vi "Main.Initialize DTC FIFOs.vi"(8 "error in":errorcluster, 11 "Sim DTCs":T2 {"DM1 Ref"."Data Reference" format="%.0x"; "DM1 Enable Ref"."Data Reference" format="%.0x"; "DM2 Ref"."Data Reference" format="%.0x"; "DM2 Enable Ref"."Data Reference" format="%.0x"}) -> (0 "error out":errorcluster, 3 "Sim DTC Refs":T1 {"Data"."DM1 Ref"."Data Reference" format="%.0x"; "Data"."DM1 Enable Ref"."Data Reference" format="%.0x"; "Data"."DM2 Ref"."Data Reference" format="%.0x"; "Data"."DM2 Enable Ref"."Data Reference" format="%.0x"})   [LabVIEW 2015, in "J1939 Addon Engine.lvlib"]
uses:
  J1939 Addon Engine.lvlib
  Shared/Types/Compiled Simulated Settings.ctl
  <vilib>/NI Veristand/Custom Device API/Block Data Reference.ctl
  <vilib>/NI Veristand/Custom Device API/Data Reference.ctl
  Types/Engine.DTC Settings.ctl
  Types/Engine.DTC FIFOs.ctl
  <vilib>/NI VeriStand/Custom Device API/Custom Device API.lvlib
  Shared/J1939 Addon Shared.lvlib
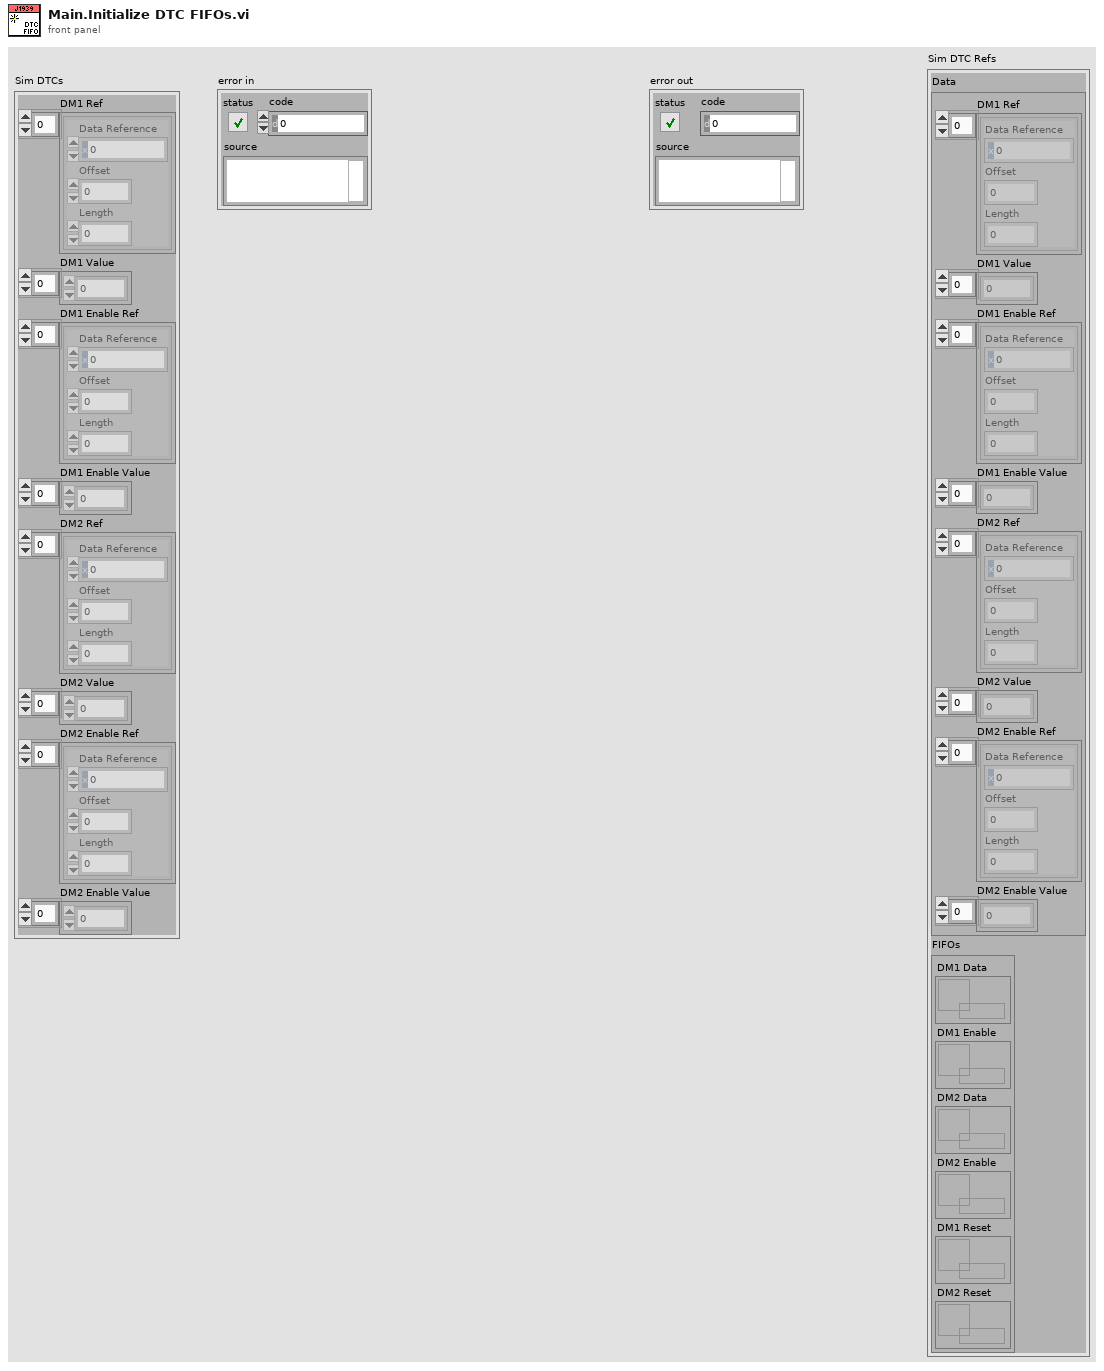
[diagram p1: front panel]
types:
  T1 = typedef "J1939 Addon Engine.lvlib/Engine.DTC Settings.ctl" = cluster{"Data":T2, "FIFOs":T5}
  T2 = typedef "J1939 Addon Shared.lvlib/Compiled Simulated Settings.ctl" = cluster{"DM1 Ref":T3[], "DM1 Value":dbl[], "DM1 Enable Ref":T3[], "DM1 Enable Value":dbl[], "DM2 Ref":T3[], "DM2 Value":dbl[], "DM2 Enable Ref":T3[], "DM2 Enable Value":dbl[]}
  T3 = typedef "Custom Device API.lvlib/Block Data Reference.ctl" = cluster{"Data Reference":T4, "Offset":u64, "Length":u64}
  T4 = typedef "Custom Device API.lvlib/Data Reference.ctl" = i32
  T5 = typedef "J1939 Addon Engine.lvlib/Engine.DTC FIFOs.ctl" = cluster{"DM1 Data":refnum<k33>, "DM1 Enable":refnum<k33>, "DM2 Data":refnum<k33>, "DM2 Enable":refnum<k33>, "DM1 Reset":refnum<k33>, "DM2 Reset":refnum<k33>}
  T6 = cluster{"read mode":enum16{"polling", "blocking"}, "write mode":enum16{"polling", "blocking"}}
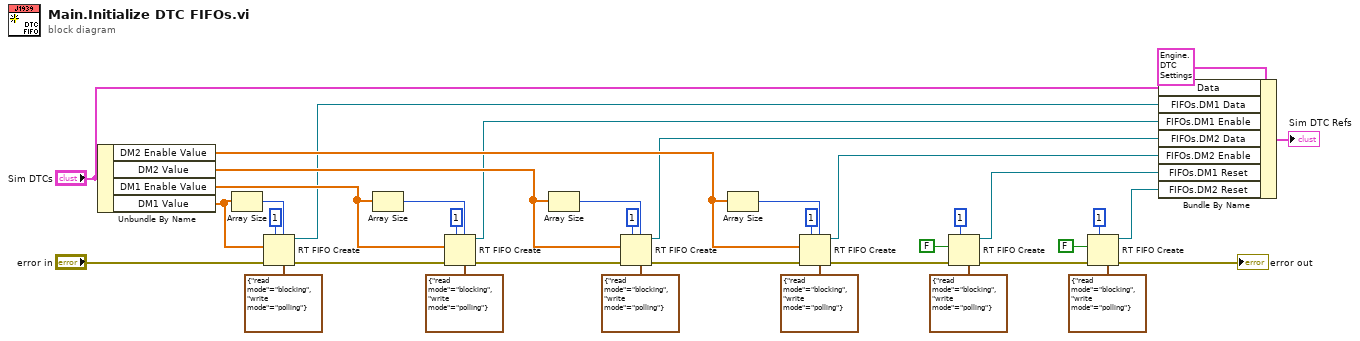
[diagram p0: block diagram]
diagram:
  n1 = Unbundle By Name("Sim DTCs") -> ("DM2 Enable Value"=w19:dbl[], "DM2 Value"=w20:dbl[], "DM1 Enable Value"=w21:dbl[], "DM1 Value"=w22:dbl[])
  n2 = Array Size(array=w22) -> (size(s)=w35:i32)
  n3 = RT FIFO Create(1:w22, 3:"error in", 4:u32 1 ("size (10)"), 6:w35, 7:T6 {"read mode"=enum."blocking", "write mode"=enum."polling"} ("r/w modes (polling,polling)")) -> (8:w18:refnum<k33>, 11:w25:errorcluster)  [unwired: 3 in, 1 out]
  n4 = Array Size(array=w21) -> (size(s)=w34:i32)
  n5 = RT FIFO Create(1:w21, 3:w25, 4:u32 1 ("size (10)"), 6:w34, 7:T6 {"read mode"=enum."blocking", "write mode"=enum."polling"} ("r/w modes (polling,polling)")) -> (8:w17:refnum<k33>, 11:w24:errorcluster)  [unwired: 3 in, 1 out]
  n6 = Array Size(array=w20) -> (size(s)=w29:i32)
  n7 = RT FIFO Create(1:w20, 3:w24, 4:u32 1 ("size (10)"), 6:w29, 7:T6 {"read mode"=enum."blocking", "write mode"=enum."polling"} ("r/w modes (polling,polling)")) -> (8:w16:refnum<k33>, 11:w23:errorcluster)  [unwired: 3 in, 1 out]
  n8 = Array Size(array=w19) -> (size(s)=w28:i32)
  n9 = RT FIFO Create(1:w19, 3:w23, 4:u32 1 ("size (10)"), 6:w28, 7:T6 {"read mode"=enum."blocking", "write mode"=enum."polling"} ("r/w modes (polling,polling)")) -> (8:w15:refnum<k33>, 11:w12:errorcluster)  [unwired: 3 in, 1 out]
  n10 = RT FIFO Create(1:FALSE, 3:w12, 4:u32 1 ("size (10)"), 7:T6 {"read mode"=enum."blocking", "write mode"=enum."polling"} ("r/w modes (polling,polling)")) -> (8:w6:refnum<k33>, 11:w7:errorcluster)  [unwired: 4 in, 1 out]
  n11 = RT FIFO Create(1:FALSE, 3:w7, 4:u32 1 ("size (10)"), 7:T6 {"read mode"=enum."blocking", "write mode"=enum."polling"} ("r/w modes (polling,polling)")) -> (8:w5:refnum<k33>, 11:→"error out":errorcluster)  [unwired: 4 in, 1 out]
  n12 = Bundle By Name(cluster=T1 {"Data"={"DM1 Ref"=[], "DM1 Value"=[], "DM1 Enable Ref"=[], "DM1 Enable Value"=[], "DM2 Ref"=[], "DM2 Value"=[], "DM2 Enable Ref"=[], "DM2 Enable Value"=[]}, "FIFOs"={"DM1 Data"=refnum, "DM1 Enable"=refnum, "DM2 Data"=refnum, "DM2 Enable"=refnum, "DM1 Reset"=refnum, "DM2 Reset"=refnum}}, "Data"="Sim DTCs", "FIFOs.DM1 Data"=w18, "FIFOs.DM1 Enable"=w17, "FIFOs.DM2 Data"=w16, "FIFOs.DM2 Enable"=w15, "FIFOs.DM1 Reset"=w6, "FIFOs.DM2 Reset"=w5) -> (→"Sim DTC Refs":T1)
